vi "swerveImmForAuto.vi"(8 "ScaleSpeed":dbl=0.5, 9 "x2":dbl, 10 "y1":dbl, 11 "x1":dbl) -> ()   [LabVIEW 2020]
uses:
  <vilib>/Rock Robotics/WPI/ThirdParty/Sensors/navX/_TypeDefs/FRIC_navX_DeviceNumbersTypeDef.ctl
  <vilib>/addons/control/pid/NI_PID_pid.lvlib
  <vilib>/addons/control/pid/pid.llb/PID (DBL).vi
  <vilib>/Rock Robotics/WPI/ThirdParty/Phoenix-LabVIEW/CANCoder/Get/CTRE_Phoenix_CANcoder_GetSensorData.vi
  <vilib>/Rock Robotics/WPI/ThirdParty/REV Robotics/REVLib/Typedef/Spark MAX Control Type.ctl
panel:
  in  "dt (s)":dbl=-1.0 format="%.3f"
  in  "PID gains 2":T1={"proportional gain (Kc)"=0.004667, "integral time (Ti, min)"=0.013, "derivative time (Td, min)"=0.0} {"derivative time (Td, min)" format="%.10f"; "integral time (Ti, min)" format="%.10f"; "proportional gain (Kc)" format="%.10f"}
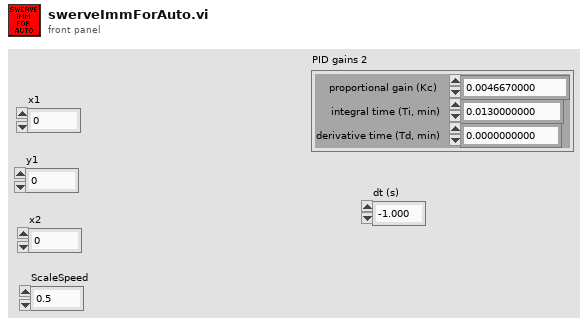
[diagram p1: front panel]
types:
  T1 = cluster{"proportional gain (Kc)":dbl, "integral time (Ti, min)":dbl, "derivative time (Td, min)":dbl}
  T2 = typedef "Spark MAX Control Type.ctl" = enum16{"Percent VBus", "Voltage", "Velocity", "Position", "Smart Motion", "Current", "Smart Velocity"}
  T3 = typedef "FRIC_navX_DeviceNumbersTypeDef.ctl" = enum16{"Dev0", "Dev1", "Dev2", "Dev3"}
  T4 = cluster{"Yaw":dbl, "Roll":dbl, "Pitch":dbl, "Heading":dbl, "Fused Heading":dbl}
  T5 = typedef "CTRE_Phoenix_CANcoder_DeviceRef.ctl" = cluster{"DeviceStatus":errorcluster, "Device Number":u8, "Handle":u64, "UsageFrame":u32, "Library Path":path}
  T6 = typedef "WPI_MotorControlDeviceRef.ctl" = cluster{"DeviceStatus":errorcluster, "Type":T7, "PWM":cluster{"PWM Channel":T8, "DeadBand":T9}, "CAN":cluster{"Device Number":u8, "SetOutput VI Ref":variant, "GetOutput VI Ref":variant, "Enable VI Ref":variant, "Disable VI Ref":variant, "Data":variant}, "Invert":bool, "DIO PWM":cluster{"PWM \"Enable\" Channel":T8, "DIOChannel":T10, "PWM Rate":dbl}}
  T7 = typedef "WPI_MotorControlType.ctl" = enum16{"PWM", "CAN", "DIO PWM"}
  T8 = typedef "FPGA_DIOPWMChannel.ctl" = enum8{"PWM 0", "PWM 1", "PWM 2", "PWM 3", "PWM 4", "PWM 5", "PWM 6", "PWM 7", "PWM 8", "PWM 9", "PWM MXP 0", "PWM MXP 1", "PWM MXP 2", "PWM MXP 3", "PWM MXP 4", "PWM MXP 5", "PWM MXP 6", "PWM MXP 7", "PWM MXP 8", "PWM MXP 9", "Invalid"}
  T9 = typedef "WPI_PWMDeadband.ctl" = cluster{"Name":string, "maxPositivePwm":i32, "minPositivePwm":i32, "centerPwm":i32, "maxNegativePwm":i32, "minNegativePwm":i32, "angularRange":u16}
  T10 = typedef "FPGA_DIOChannel.ctl" = enum8{"DIO 0", "DIO 1", "DIO 2", "DIO 3", "DIO 4", "DIO 5", "DIO 6", "DIO 7", "DIO 8", "DIO 9", "DIO MXP 0", "DIO MXP 1", "DIO MXP 2", "DIO MXP 3", "DIO MXP 4", "DIO MXP 5", "DIO MXP 6", "DIO MXP 7", "DIO MXP 8", "DIO MXP 9", "DIO MXP 10", "DIO MXP 11", "DIO MXP 12", "DIO MXP 13", "DIO MXP 14", "DIO MXP 15", "SPI Port CS1", "SPI Port CS2", "SPI Port CS3", "SPI Port MISO", "SPI Port MOSI", "Invalid"}
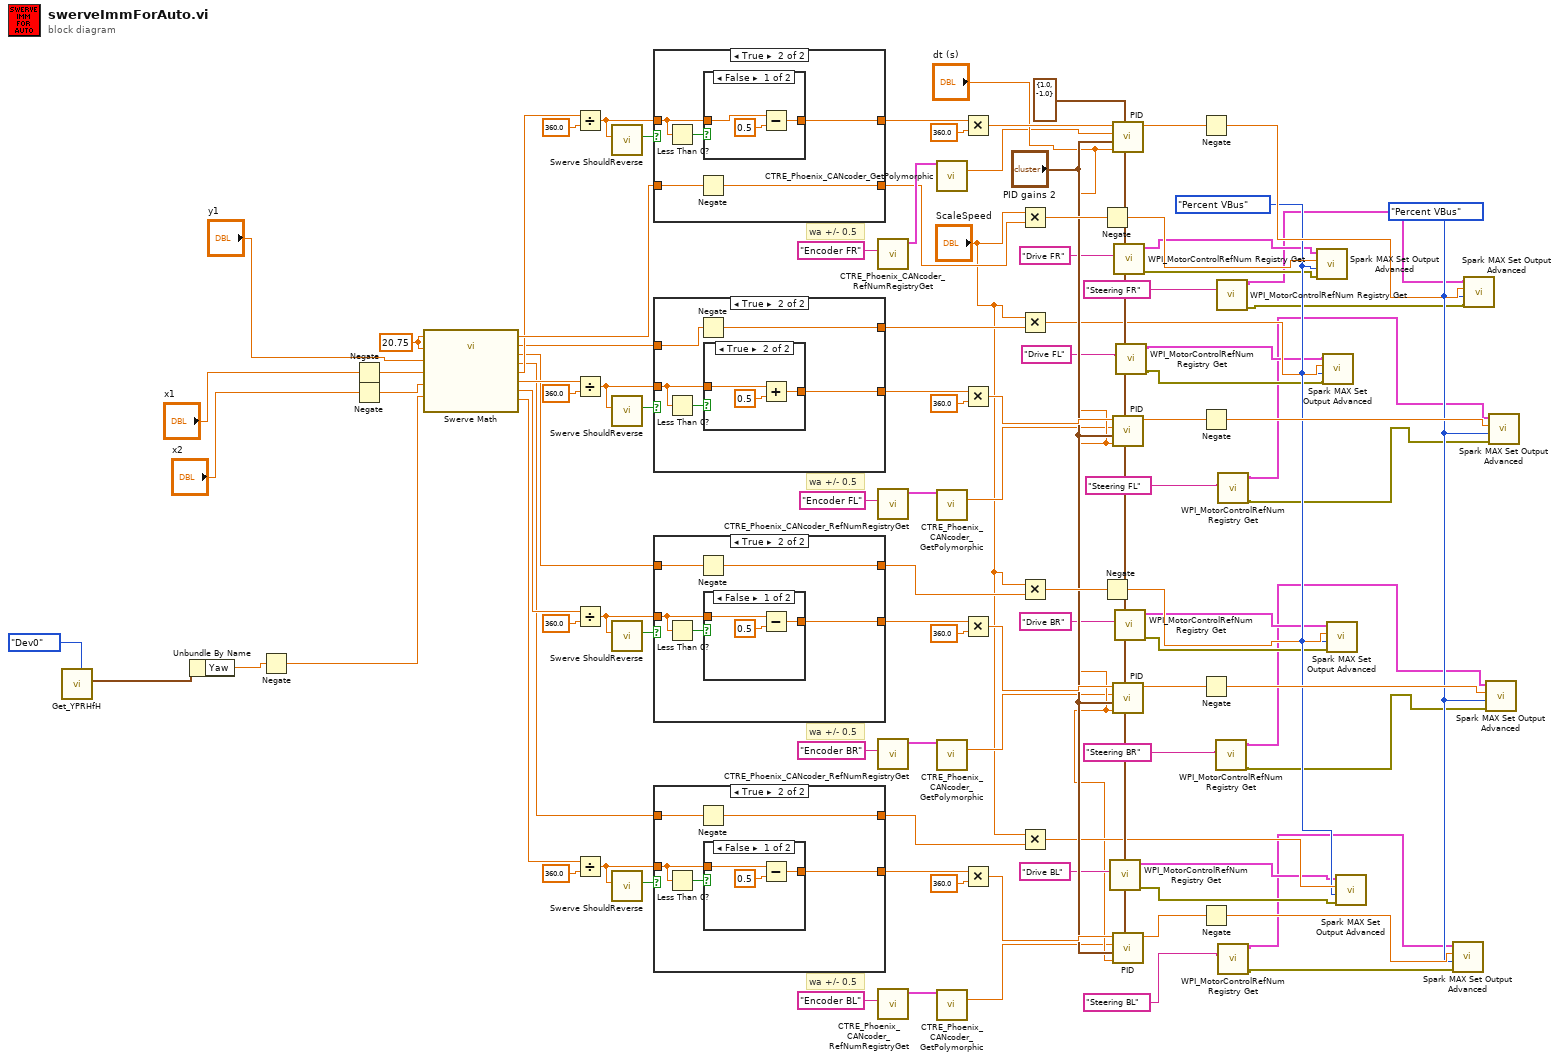
[diagram p0: block diagram]
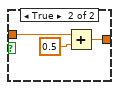
[diagram p3: hidden frame]
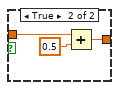
[diagram p5: hidden frame]
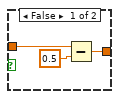
[diagram p7: hidden frame]
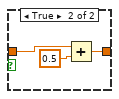
[diagram p9: hidden frame]
diagram:
  w37 = Spark_MAX_Control_Type."Percent VBus" ("Control Mode")
  w42 = Spark_MAX_Control_Type."Percent VBus" ("Control Mode")
  w47 = cluster{"output high":dbl, "output low":dbl} {"output high"=1.0, "output low"=-1.0} ("output range")
  w99 = 20.75 ("Trackwidth (W)")
  (unwired) FRIC_navX_DeviceNumbersTypeDef."Dev0" ("Device Number")
  # "wa +/- 0.5"
  # "wa +/- 0.5"
  # "wa +/- 0.5"
  # "wa +/- 0.5"
  n1 = call <vilib>:"Get_YPRHfH.vi"("Device Number"=FRIC_navX_DeviceNumbersTypeDef."Dev0") -> ("YRPHfH"=w101:T4)  [unwired: 10 in]
  n2 = Unbundle By Name(w101) -> ("Yaw"=w100:dbl)
  n3 = Negate(x=w100) -> (-x=w2:dbl)
  n4 = Negate(x="x1") -> (-x=w4:dbl)
  n5 = Negate(x="x2") -> (-x=w3:dbl)
  n6 = call "Swerve Math.vi"("Trackwidth (W)"=w99, "Wheelbase (L)"=w99, "Y -FWD"="y1", "X1 STR"=w4, "X2 RCW"=w3, "Gyro Angle in degrees"=w2) -> ("wa3"=w51:dbl, "wa4"=w49:dbl, "ws1"=w56:dbl, "ws2"=w54:dbl, "ws3"=w52:dbl, "ws4"=w50:dbl, "wa2"=w53:dbl, "wa1"=w55:dbl)  [unwired: 2 in]
  n7 = Divide(x=w55, y=360.0) -> (x/y=w93:dbl)
  n8 = Divide(x=w53, y=360.0) -> (x/y=w82:dbl)
  n9 = Divide(x=w51, y=360.0) -> (x/y=w72:dbl)
  n10 = Divide(x=w49, y=360.0) -> (x/y=w61:dbl)
  n11 = call "Swerve ShouldReverse.vi"("wa in"=w93) -> ("shouldReverse out"=w94:bool)  [unwired: 10 in]
  n12 = call "Swerve ShouldReverse.vi"("wa in"=w82) -> ("shouldReverse out"=w83:bool)  [unwired: 10 in]
  n13 = call "Swerve ShouldReverse.vi"("wa in"=w72) -> ("shouldReverse out"=w73:bool)  [unwired: 10 in]
  n14 = call "Swerve ShouldReverse.vi"("wa in"=w61) -> ("shouldReverse out"=w62:bool)  [unwired: 10 in]
  n15 = case shown="True" w94 {
    tunnel: w56 -> [w104 w105]
    tunnel: w93 -> [w103 w108]
    tunnel: [w104 w106] -> w92
    tunnel: [w103 w107] -> w91
    frame False {
    }
    frame True {
      n16 = Less Than 0?(x=w108) -> (x < 0?=w109:bool)
      n17 = Negate(x=w105) -> (-x=w106:dbl)
      n18 = case shown="False" w109 {
        tunnel: w108 -> [w111 w114]
        tunnel: [w110 w113] -> w107
        frame False {
          n19 = Subtract(x=w111, y=0.5) -> (x-y=w110:dbl)
        }
        frame True {
          n20 = Add(x=w114, y=0.5) -> (x+y=w113:dbl)
        }
      }
    }
  }
  n21 = case shown="True" w83 {
    tunnel: w54 -> [w117 w118]
    tunnel: w82 -> [w116 w121]
    tunnel: [w117 w119] -> w81
    tunnel: [w116 w120] -> w80
    frame False {
    }
    frame True {
      n22 = Less Than 0?(x=w121) -> (x < 0?=w122:bool)
      n23 = Negate(x=w118) -> (-x=w119:dbl)
      n24 = case shown="True" w122 {
        tunnel: w121 -> [w124 w127]
        tunnel: [w123 w126] -> w120
        frame False {
          n25 = Subtract(x=w124, y=0.5) -> (x-y=w123:dbl)
        }
        frame True {
          n26 = Add(x=w127, y=0.5) -> (x+y=w126:dbl)
        }
      }
    }
  }
  n27 = case shown="True" w73 {
    tunnel: w52 -> [w130 w131]
    tunnel: w72 -> [w129 w134]
    tunnel: [w130 w132] -> w71
    tunnel: [w129 w133] -> w70
    frame False {
    }
    frame True {
      n28 = Less Than 0?(x=w134) -> (x < 0?=w135:bool)
      n29 = Negate(x=w131) -> (-x=w132:dbl)
      n30 = case shown="False" w135 {
        tunnel: w134 -> [w137 w140]
        tunnel: [w136 w139] -> w133
        frame False {
          n31 = Subtract(x=w137, y=0.5) -> (x-y=w136:dbl)
        }
        frame True {
          n32 = Add(x=w140, y=0.5) -> (x+y=w139:dbl)
        }
      }
    }
  }
  n33 = case shown="True" w62 {
    tunnel: w50 -> [w143 w144]
    tunnel: w61 -> [w142 w147]
    tunnel: [w143 w145] -> w60
    tunnel: [w142 w146] -> w59
    frame False {
    }
    frame True {
      n34 = Less Than 0?(x=w147) -> (x < 0?=w148:bool)
      n35 = Negate(x=w144) -> (-x=w145:dbl)
      n36 = case shown="False" w148 {
        tunnel: w147 -> [w150 w153]
        tunnel: [w149 w152] -> w146
        frame False {
          n37 = Subtract(x=w150, y=0.5) -> (x-y=w149:dbl)
        }
        frame True {
          n38 = Add(x=w153, y=0.5) -> (x+y=w152:dbl)
        }
      }
    }
  }
  n39 = call <vilib>:"CTRE_Phoenix_CANcoder_RefNumRegistryGet.vi"("refnum name"="Encoder FR") -> ("CTRE_CANcoder_DeviceRef"=w97:T5)  [unwired: 9 in, 1 out]
  n40 = call <vilib>:"CTRE_Phoenix_CANcoder_RefNumRegistryGet.vi"("refnum name"="Encoder FL") -> ("CTRE_CANcoder_DeviceRef"=w86:T5)  [unwired: 9 in, 1 out]
  n41 = call <vilib>:"CTRE_Phoenix_CANcoder_RefNumRegistryGet.vi"("refnum name"="Encoder BR") -> ("CTRE_CANcoder_DeviceRef"=w76:T5)  [unwired: 9 in, 1 out]
  n42 = call <vilib>:"CTRE_Phoenix_CANcoder_RefNumRegistryGet.vi"("refnum name"="Encoder BL") -> ("CTRE_CANcoder_DeviceRef"=w65:T5)  [unwired: 9 in, 1 out]
  n43 = call-poly <vilib>:"CTRE_Phoenix_CANcoder_GetPolymorphic.vi"("CTRE_CANcoder_DeviceRef"=w97) -> ("Position"=w9:dbl)  [unwired: 10 in, 4 out]
  n44 = call-poly <vilib>:"CTRE_Phoenix_CANcoder_GetPolymorphic.vi"("CTRE_CANcoder_DeviceRef"=w86) -> ("Position"=w10:dbl)  [unwired: 10 in, 4 out]
  n45 = call-poly <vilib>:"CTRE_Phoenix_CANcoder_GetPolymorphic.vi"("CTRE_CANcoder_DeviceRef"=w76) -> ("Position"=w11:dbl)  [unwired: 10 in, 4 out]
  n46 = call-poly <vilib>:"CTRE_Phoenix_CANcoder_GetPolymorphic.vi"("CTRE_CANcoder_DeviceRef"=w65) -> ("Position"=w8:dbl)  [unwired: 10 in, 4 out]
  n47 = Multiply(x=w91, y=360.0) -> (x*y=w90:dbl)
  n48 = Multiply(x=w80, y=360.0) -> (x*y=w79:dbl)
  n49 = Multiply(x=w70, y=360.0) -> (x*y=w69:dbl)
  n50 = Multiply(x=w59, y=360.0) -> (x*y=w58:dbl)
  n51 = Multiply(x="ScaleSpeed", y=w92) -> (x*y=w88:dbl)
  n52 = Multiply(x="ScaleSpeed", y=w81) -> (x*y=w40:dbl)
  n53 = Multiply(x="ScaleSpeed", y=w71) -> (x*y=w67:dbl)
  n54 = Multiply(x="ScaleSpeed", y=w60) -> (x*y=w38:dbl)
  n55 = Negate(x=w88) -> (-x=w41:dbl)
  n56 = Negate(x=w67) -> (-x=w39:dbl)
  n57 = call <vilib>:"WPI_MotorControlRefNum Registry Get.vi"("refnum name"="Drive BL") -> ("error out"=w17:errorcluster, "MotorControlDevRef"=w18:T6)  [unwired: 9 in]
  n58 = call-poly <vilib>:"PID.vi"("output range"=w47, "dt (s)"="dt (s)", "PID gains"="PID gains 2", "process variable"=w9, "setpoint"=w90) -> ("output"=w98:dbl)  [unwired: 5 in, 1 out]
  n59 = call-poly <vilib>:"PID.vi"("output range"=w47, "dt (s)"="dt (s)", "PID gains"="PID gains 2", "process variable"=w10, "setpoint"=w79) -> ("output"=w87:dbl)  [unwired: 5 in, 1 out]
  n60 = call-poly <vilib>:"PID.vi"("output range"=w47, "dt (s)"="dt (s)", "PID gains"="PID gains 2", "process variable"=w11, "setpoint"=w69) -> ("output"=w77:dbl)  [unwired: 5 in, 1 out]
  n61 = call-poly <vilib>:"PID.vi"("output range"=w47, "dt (s)"="dt (s)", "PID gains"="PID gains 2", "process variable"=w8, "setpoint"=w58) -> ("output"=w66:dbl)  [unwired: 5 in, 1 out]
  n62 = call <vilib>:"WPI_MotorControlRefNum Registry Get.vi"("refnum name"="Drive FR") -> ("error out"=w34:errorcluster, "MotorControlDevRef"=w35:T6)  [unwired: 9 in]
  n63 = call <vilib>:"WPI_MotorControlRefNum Registry Get.vi"("refnum name"="Drive BR") -> ("error out"=w22:errorcluster, "MotorControlDevRef"=w23:T6)  [unwired: 9 in]
  n64 = call <vilib>:"WPI_MotorControlRefNum Registry Get.vi"("refnum name"="Drive FL") -> ("error out"=w28:errorcluster, "MotorControlDevRef"=w29:T6)  [unwired: 9 in]
  n65 = Negate(x=w98) -> (-x=w46:dbl)
  n66 = Negate(x=w87) -> (-x=w45:dbl)
  n67 = Negate(x=w77) -> (-x=w44:dbl)
  n68 = Negate(x=w66) -> (-x=w43:dbl)
  n69 = call <vilib>:"WPI_MotorControlRefNum Registry Get.vi"("refnum name"="Steering BR") -> ("error out"=w20:errorcluster, "MotorControlDevRef"=w21:T6)  [unwired: 9 in]
  n70 = call <vilib>:"WPI_MotorControlRefNum Registry Get.vi"("refnum name"="Steering FR") -> ("error out"=w31:errorcluster, "MotorControlDevRef"=w32:T6)  [unwired: 9 in]
  n71 = call <vilib>:"WPI_MotorControlRefNum Registry Get.vi"("refnum name"="Steering FL") -> ("error out"=w25:errorcluster, "MotorControlDevRef"=w26:T6)  [unwired: 9 in]
  n72 = call <vilib>:"WPI_MotorControlRefNum Registry Get.vi"("refnum name"="Steering BL") -> ("error out"=w14:errorcluster, "MotorControlDevRef"=w15:T6)  [unwired: 9 in]
  n73 = call <vilib>:"Spark MAX Set Output Advanced.vi"("error in (no error)"=w34, "Control Mode"=w37, "Setpoint"=w41, "MotorControlDevRef"=w35) -> ()  [unwired: 6 in, 2 out]
  n74 = call <vilib>:"Spark MAX Set Output Advanced.vi"("error in (no error)"=w28, "Control Mode"=w37, "Setpoint"=w40, "MotorControlDevRef"=w29) -> ()  [unwired: 6 in, 2 out]
  n75 = call <vilib>:"Spark MAX Set Output Advanced.vi"("error in (no error)"=w22, "Control Mode"=w37, "Setpoint"=w39, "MotorControlDevRef"=w23) -> ()  [unwired: 6 in, 2 out]
  n76 = call <vilib>:"Spark MAX Set Output Advanced.vi"("error in (no error)"=w17, "Control Mode"=w37, "Setpoint"=w38, "MotorControlDevRef"=w18) -> ()  [unwired: 6 in, 2 out]
  n77 = call <vilib>:"Spark MAX Set Output Advanced.vi"("error in (no error)"=w14, "Control Mode"=w42, "Setpoint"=w43, "MotorControlDevRef"=w15) -> ()  [unwired: 6 in, 2 out]
  n78 = call <vilib>:"Spark MAX Set Output Advanced.vi"("error in (no error)"=w31, "Control Mode"=w42, "Setpoint"=w46, "MotorControlDevRef"=w32) -> ()  [unwired: 6 in, 2 out]
  n79 = call <vilib>:"Spark MAX Set Output Advanced.vi"("error in (no error)"=w20, "Control Mode"=w42, "Setpoint"=w44, "MotorControlDevRef"=w21) -> ()  [unwired: 6 in, 2 out]
  n80 = call <vilib>:"Spark MAX Set Output Advanced.vi"("error in (no error)"=w25, "Control Mode"=w42, "Setpoint"=w45, "MotorControlDevRef"=w26) -> ()  [unwired: 6 in, 2 out]
